vi "Access Tests.vi"() -> ()   [LabVIEW 2020]
uses:
  FGV Map/Controls/FGV Map Core State.ctl
  FGV Map/Get Data/FGV Map Get Data (Bool).vi
  FGV Map/Get Data/FGV Map Get Data (Variant).vi
  FGV Map/Get Data/FGV Map Get Data (I32).vi
  FGV Map.lvlib
panel:
  out "Instance Out":map{string, variant}(c390)
  out "Data Not Found ? 5":bool
  out "Data Out 3":bool
  out "Data Not Found ? 4":bool
  out "Data Out 2":bool
  out "Instance Created ? 4":bool
  out "Data Overwritten ? 4":bool
  out "Data Not Found ? 3":bool
  out "Data Not Found ? 2":bool
  out "Data Not Found ?":bool
  out "Instance Created ? 3":bool
  out "Data Overwritten ? 3":bool
  out "Instance Created ? 2":bool
  out "Data Overwritten ? 2":bool
  out "Instance Created ?":bool
  out "Data Overwritten ?":bool
  out "data":waveform(dbl)
  out "Data Out":i32
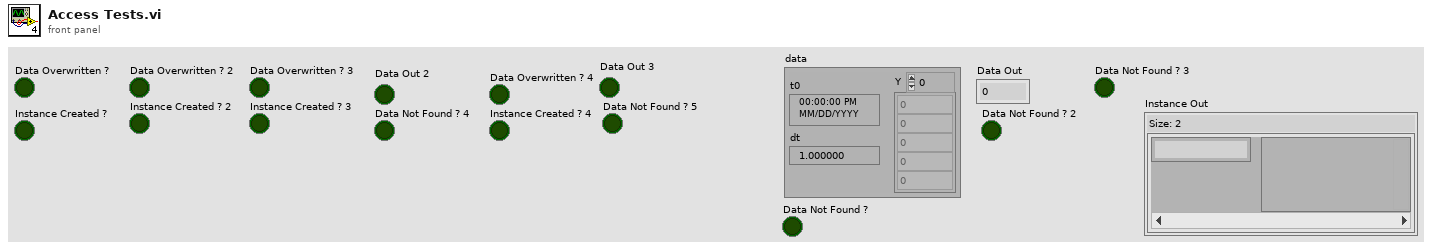
[diagram p1: front panel]
types:
  T1 = typedef "FGV Map.lvlib/FGV Map Core State.ctl" = enum16{"Init", "Set Instance (Unlock)", "Get Instance", "Get Instance (Lock)", "Unlock", "Get All Instances", "Delete Instance"}
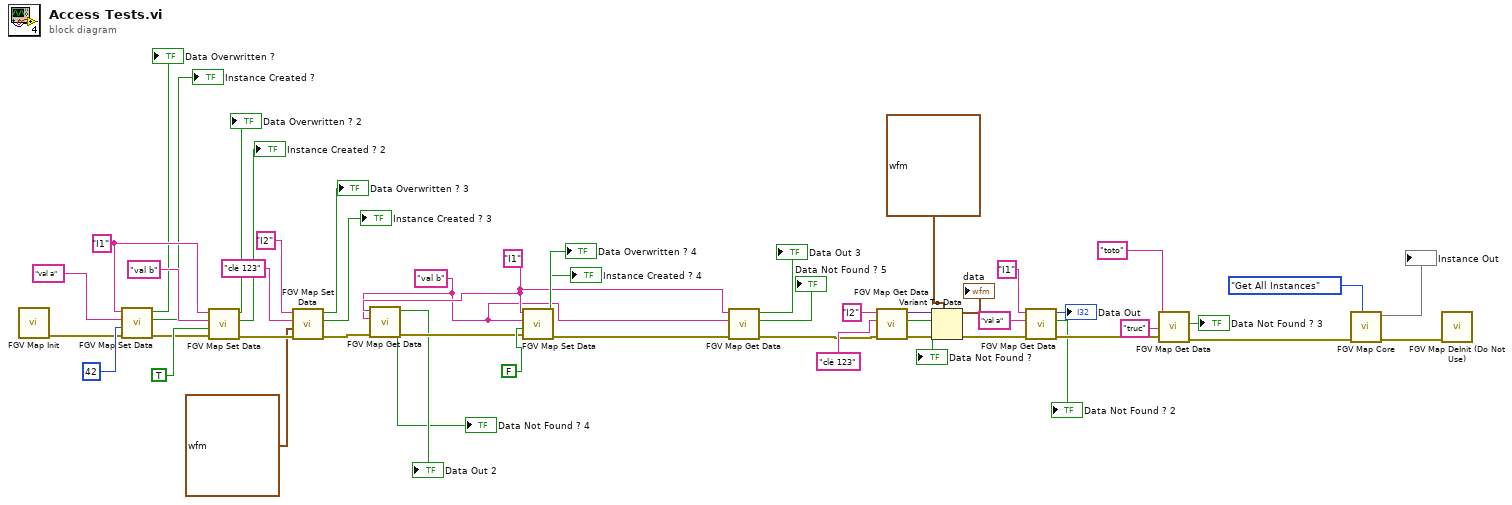
[diagram p0: block diagram]
diagram:
  w8 = "val b" ("Data Key")
  w9 = "I1" ("Instance Key")
  w50 = "I1" ("Instance Key")
  n1 = call "FGV Map Init.vi"() -> ("error out"=w5:errorcluster)  [unwired: 11 in]
  n2 = call "FGV Map Set Data.vi"("error in (no error)"=w5, "Data In"=42, "Data Key"="val a", "Instance Key"=w50) -> ("error out"=w45:errorcluster, "Instance Created ?"=→"Instance Created ?":bool, "Data Overwritten ?"=→"Data Overwritten ?":bool)  [unwired: 5 in]
  n3 = call "FGV Map Set Data.vi"("error in (no error)"=w45, "Data In"=TRUE, "Data Key"="val b", "Instance Key"=w50) -> ("error out"=w44:errorcluster, "Instance Created ?"=→"Instance Created ? 2":bool, "Data Overwritten ?"=→"Data Overwritten ? 2":bool)  [unwired: 5 in]
  n4 = call "FGV Map Set Data.vi"("error in (no error)"=w44, "Data In"=waveform(dbl) {"t0"=timestamp(3061148400 s since 1904-01-01), "dt"=1.0, "Y"=[1.0, 2.0, 3.0]} ("Waveform"), "Data Key"="clé 123", "Instance Key"="I2") -> ("error out"=w15:errorcluster, "Instance Created ?"=→"Instance Created ? 3":bool, "Data Overwritten ?"=→"Data Overwritten ? 3":bool)  [unwired: 5 in]
  n5 = call-poly "FGV Map Get Data.vi"("error in (no error)"=w15, "Data Key"=w8, "Instance Key"=w9) -> ("error out"=w14:errorcluster, "Data Not Found ?"=→"Data Not Found ? 4":bool, "Data Out"=→"Data Out 2":bool)  [unwired: 6 in]
  n6 = call "FGV Map Set Data.vi"("error in (no error)"=w14, "Data In"=FALSE, "Data Key"=w8, "Instance Key"=w9) -> ("error out"=w11:errorcluster, "Instance Created ?"=→"Instance Created ? 4":bool, "Data Overwritten ?"=→"Data Overwritten ? 4":bool)  [unwired: 5 in]
  n7 = call-poly "FGV Map Get Data.vi"("error in (no error)"=w11, "Data Key"=w8, "Instance Key"=w9) -> ("error out"=w10:errorcluster, "Data Not Found ?"=→"Data Not Found ? 5":bool, "Data Out"=→"Data Out 3":bool)  [unwired: 6 in]
  n8 = call-poly "FGV Map Get Data.vi"("error in (no error)"=w10, "Data Key"="clé 123", "Instance Key"="I2") -> ("error out"=w42:errorcluster, "Data Not Found ?"=→"Data Not Found ?":bool, "Data Out"=w41:variant)  [unwired: 6 in]
  n9 = Variant To Data(error in=w42, type=waveform(dbl) {"t0"=timestamp(0 s since 1904-01-01), "dt"=1.0, "Y"=[]} ("Waveform"), Variant=w41) -> (data=→"data":waveform(dbl), error out=w37:errorcluster)
  n10 = call-poly "FGV Map Get Data.vi"("error in (no error)"=w37, "Data Key"="val a", "Instance Key"="I1") -> ("error out"=w32:errorcluster, "Data Not Found ?"=→"Data Not Found ? 2":bool, "Data Out"=→"Data Out":i32)  [unwired: 6 in]
  n11 = call-poly "FGV Map Get Data.vi"("error in (no error)"=w32, "Data Key"="truc", "Instance Key"="toto") -> ("error out"=w4:errorcluster, "Data Not Found ?"=→"Data Not Found ? 3":bool)  [unwired: 6 in, 1 out]
  n12 = call "FGV Map Core.vi"("FGV State"=FGV_Map_Core_State."Get All Instances", "error in"=w4) -> ("error out"=w2:errorcluster, "Instance Out"=→"Instance Out":map{string, variant})  [unwired: 5 in, 3 out]
  n13 = call "FGV Map DeInit (Do Not Use).vi"("error in"=w2) -> ()  [unwired: 10 in, 1 out]
